vi "XLP80_Action_StartTestmode_A.vi"(8 "err in":errorcluster) -> (0 "err out":errorcluster)   [LabVIEW 2021]
uses:
  XLP80_FGlob/1886_FGlob_TDefs_Enum_FGlobItems.ctl
  XLP80_FGlob/1886_FGlob_TDefEnumCANWriteItems.ctl
  XLP80_Globals/XLP80_Globals_Referenzen.vi
  XLP80_Globals/XLP80_CAN_Globals.vi
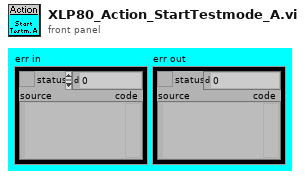
[diagram p1: front panel]
types:
  T1 = typedef "1886_FGlob_TDefs_Enum_FGlobItems.ctl" = enum16{"Put one", "Put all", "Recall one", "Recall all"}
  T2 = typedef "1886_FGlob_TDefEnumCANWriteItems.ctl" = enum16{"LV_Testmode_Select", "LV_A_71_Current_Out_Set", "LV_A_71_Voltage_In_Set", "LV_A_71_Voltage_Out_Set", "LV_H_51_STK_CellVoltages_Enable", "S80_BP_s_Taster_Start_Status"}
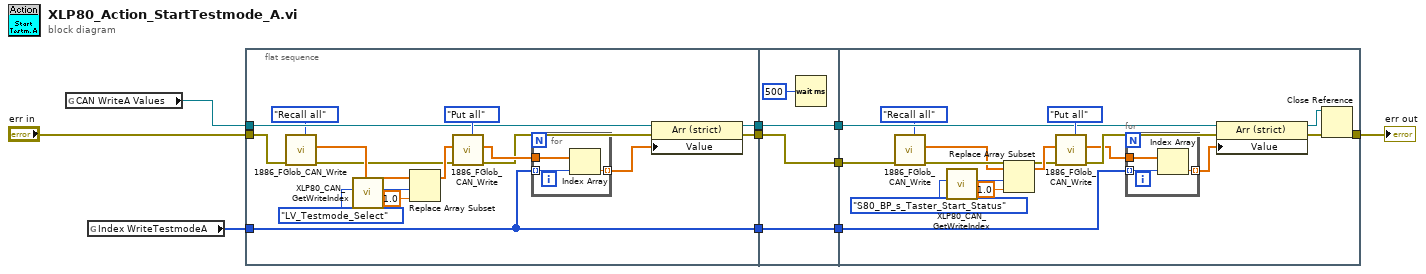
[diagram p0: block diagram]
diagram:
  n1 = global read "XLP80_Globals_Referenzen.vi" "CAN WriteA Values"() -> (w1:refnum<vi>)
  n2 = global read "XLP80_CAN_Globals.vi" "Index WriteTestmodeA"() -> (w6:i32[])
  n3 = flat-sequence {
    tunnel: "err in" -> [w16]
    tunnel: w1 -> [w24]
    tunnel: [w23] -> w10
    tunnel: [w22] -> w9
    tunnel: w6 -> [w11]
    tunnel: [w11] -> w4
    tunnel: w10 -> [w31]
    tunnel: w9 -> [w32]
    tunnel: [w32] -> w8
    tunnel: [w31] -> w5
    tunnel: w4 -> [w30]
    tunnel: [w30] -> w3
    tunnel: w8 -> [w46]
    tunnel: [w43] -> w7
    tunnel: w5 -> [w39]
    tunnel: w3 -> [w36]
    frame #0 {
      n4 = call "1886_FGlob_CAN_Write.vi"("Function (Recall One)"=1886_FGlob_TDefs_Enum_FGlobItems."Recall all", "err in"=w16) -> ("err out"=w15:errorcluster, "AO Values OUT"=w18:dbl[])  [unwired: 7 in, 1 out]
      n5 = call "XLP80_CAN_GetWriteIndex.vi"("CAN Write Items"=1886_FGlob_TDefEnumCANWriteItems."LV_Testmode_Select" ("CAN Write Items Testmode_A")) -> ("Index"=w21:i32)  [unwired: 10 in]
      n6 = Replace Array Subset(array=w18, new element=1.0 ("new element/subarray"), index=w21) -> (w17:dbl[])
      n7 = call "1886_FGlob_CAN_Write.vi"("Function (Recall One)"=1886_FGlob_TDefs_Enum_FGlobItems."Put all", "err in"=w15, "AO Values IN"=w17) -> ("err out"=w12:errorcluster, "AO Values OUT"=w14:dbl[])  [unwired: 6 in, 1 out]
      n8 = for {
        tunnel: w11 -> [w28] mode=indexing
        tunnel: w14 -> [w29]
        tunnel: [w27] -> w13 mode=indexing
        n9 = Index Array(array=w29, index=w28) -> (element=w27:dbl)
      }
      n10 = property class="Arr (strict)"(reference=w24, error in=w12, "Value"=w13) -> (reference out=w22:refnum<vi>, error out=w23:errorcluster)
    }
    frame #1 {
      n11 = Wait (ms)(milliseconds to wait=u32 500) -> ()  [unwired: 1 out]
    }
    frame #2 {
      n12 = call "1886_FGlob_CAN_Write.vi"("Function (Recall One)"=1886_FGlob_TDefs_Enum_FGlobItems."Recall all", "err in"=w39) -> ("err out"=w38:errorcluster, "AO Values OUT"=w37:dbl[])  [unwired: 7 in, 1 out]
      n13 = call "XLP80_CAN_GetWriteIndex.vi"("CAN Write Items"=1886_FGlob_TDefEnumCANWriteItems."S80_BP_s_Taster_Start_Status" ("CAN Write Items Testmode_A")) -> ("Index"=w42:i32)  [unwired: 10 in]
      n14 = Replace Array Subset(array=w37, new element=1.0 ("new element/subarray"), index=w42) -> (w49:dbl[])
      n15 = call "1886_FGlob_CAN_Write.vi"("Function (Recall One)"=1886_FGlob_TDefs_Enum_FGlobItems."Put all", "err in"=w38, "AO Values IN"=w49) -> ("err out"=w50:errorcluster, "AO Values OUT"=w35:dbl[])  [unwired: 6 in, 1 out]
      n16 = for {
        tunnel: w36 -> [w52] mode=indexing
        tunnel: w35 -> [w53]
        tunnel: [w51] -> w34 mode=indexing
        n17 = Index Array(array=w53, index=w52) -> (element=w51:dbl)
      }
      n18 = property class="Arr (strict)"(reference=w46, error in=w50, "Value"=w34) -> (reference out=w44:refnum<vi>, error out=w45:errorcluster)
      n19 = Close Reference(reference=w44, error in (no error)=w45) -> (error out=w43:errorcluster)
    }
  }
  "err out" <- w7
